vi "tcs shm put Sample Loop Time ms LV.vi"(8 "error in (no error)":errorcluster, 11 "LoopTime_ms_Ctl":cluster{"LoopTime_ms":dbl}) -> (0 "error out":errorcluster, 2 "function return":i32, 3 "LoopTime_ms_Ctl out":cluster{"LoopTime_ms":dbl})   [LabVIEW 2016, in "SALLV_tcs.lvlib"]
doc: "int tcs_shm_putSample_LoopTime_msLV(tcs_LoopTime_msLV *LoopTime_ms_Ctl );"
uses:
  SALLV_tcs.lvlib
  SALLV_tcs.so
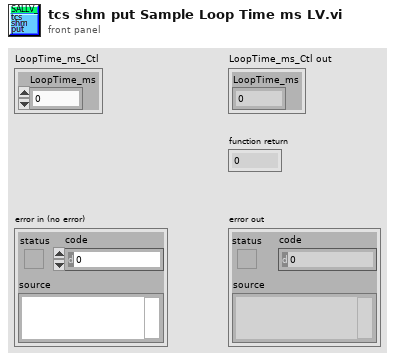
[diagram p1: front panel]
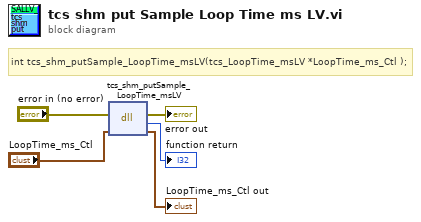
[diagram p0: block diagram]
diagram:
  # "int tcs_shm_putSample_LoopTime_msLV(tcs_LoopTime_msLV *LoopTime_ms_Ctl );"
  n1 = dll-call lib="home/plotz/SALLV_tcs/SALLV_tcs.*" fn="tcs_shm_putSample_LoopTime_msLV"(error in="error in (no error)", "LoopTime_ms_Ctl"="LoopTime_ms_Ctl") -> (error out=→"error out":errorcluster, →"function return":i32, "LoopTime_ms_Ctl"=→"LoopTime_ms_Ctl out":cluster{"LoopTime_ms":dbl})  [unwired: 2 in, 1 out]
